vi "CommandFIFO.vi"   [LabVIEW 2018]
uses:
  <vilib>/rvi/Emulation/niFpgaGetClockAttributes.vi
  <vilib>/rvi/Emulation/niFpgaSctlEmulationGetInTimedLoop.vi
  <vilib>/rvi/Emulation/niFpgaEmulationReportErrorSimple.vi
  <vilib>/rvi/interface/RandomDataEmulation/niFpgaRandomDataHandleErrors.vi
  <vilib>/rvi/DataTransferAndStorage/Container/Common/niFpgaContainerExecOnDevCompGetState.vi
  <vilib>/rvi/Emulation/niFpgaEmulationIsFPGAContextNoSignature.vi
  <vilib>/rvi/errors/niFpgaSetErrorForExecOnDevCompSimple.vi
  <vilib>/rvi/eio/common/nirviEmuReportErrorAndStop.vi
  <vilib>/rvi/DataTransferAndStorage/Container/Common/niFpgaContainerGetUniqueNameForEmu.vi
  <vilib>/rvi/FIFO/Fifo_Resource/nirvififoEmulationSetSize.vi
  <vilib>/rvi/FIFO/Fifo_Resource/nirviFifoEmulationQueueMgr.vi
  <instcachedir>/0/nirviFifoEmulationQueueMgr_E5CAEC123FF24DC58D834DCA3CDAA9B5.lvgen/nirviFifoEmulationQueueMgr_E5CAEC123FF24DC58D834DCA3CDAA9B5_012.vi
  <vilib>/rvi/FIFO/Fifo_Resource/nirvififoEmulationDetermineInputValidOut.vi
  <vilib>/rvi/FIFO/Fifo_Resource/nirvififoEmulationCreateLock.vi
  <vilib>/rvi/Emulation/niFpgaProcessEmulError.vi
  <vilib>/rvi/FIFO/Fifo_Resource/nirvififoEmulationObtainLock.vi
  <vilib>/rvi/FIFO/Fifo_Resource/nirvififoEmulationReleaseLock.vi
  <vilib>/rvi/occurrence/nirviWaitOnOccurrenceBase.vi
  <vilib>/rvi/errors/nirviReportUnexpectedCaseInternalError.vi
  <vilib>/rvi/errors/nirviReportUnexpectedCaseInternalError (U32).vi
  <vilib>/Utility/error.llb/Clear Errors.vi
  <vilib>/rvi/Memory/Memory_Emulation/niFpgaMemoryEmulationCacheClearOnFirstRun.vi
  <vilib>/rvi/Memory/Memory_Emulation/nirvimemoryEmulationManagerCache_MakeExclusive.vi
  <vilib>/rvi/Memory/Memory_Emulation/niFpgaMemoryEmulationValidateCache.vi
  <vilib>/rvi/Memory/Memory_Emulation/nirvimemoryEmulationManagerCache_InsertValue.vi
  <vilib>/rvi/Memory/Memory_Emulation/nirvimemoryEmulationManagerCache_ReleaseExclusive.vi
  <vilib>/rvi/Memory/Memory_Emulation/nirvimemoryEmulationManagerCache_GetValue.vi
  <vilib>/rvi/Memory/Memory_Emulation/nirvimemoryEmulationManagerCache_SetValue.vi
  <instcachedir>/0/nirviFifoEmulationQueueMgr_E5CAEC123FF24DC58D834DCA3CDAA9B5.lvgen/nirviFifoEmulationQueueMgr_E5CAEC123FF24DC58D834DCA3CDAA9B5_017.vi
  <vilib>/rvi/Emulation/niFpgaCriticalErrorInLSC.vi
  <vilib>/rvi/DataTransferAndStorage/Container/XNode/niFpgaContainer.xnode
  <vilib>/rvi/interface/RandomDataEmulation/nirviRandomDataFpgaReadWriteTemplate.vi
  <vilib>/rvi/FIFO/Fifo_Resource/niFpgaFifoEmulationRefIn.vi
  <vilib>/rvi/DataTransferAndStorage/Register/Emulation/niFpgaRegisterEmulation.vi
  <vilib>/rvi/FIFO/Fifo_Resource/nirvififoEmulationWrite.vi
types:
  T1 = typedef "Addresses.ctl" = enum8{"NA", "Accelerometers", "Timestamp", "ChasisTemperature"}
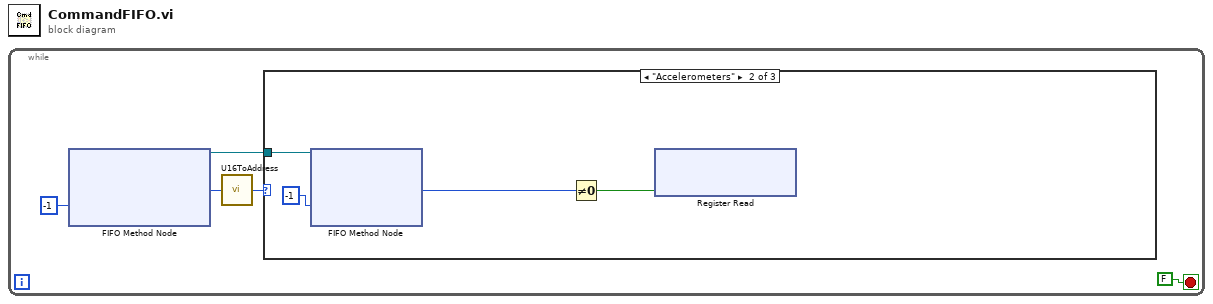
[diagram p0: block diagram]
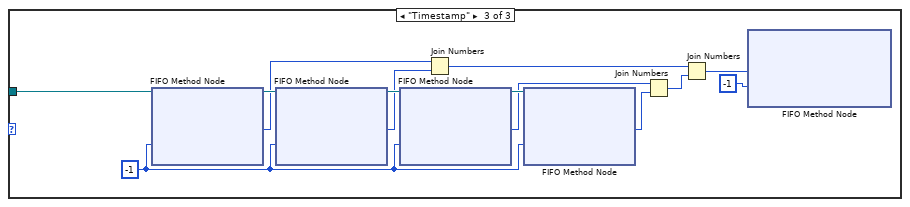
[diagram p3: hidden frame]
diagram:
  n1 = while {
    stop <- FALSE stop-if-true
    n2 = xnode ("FIFO Method Node")("Timeout"=-1) -> ("Element"=w3:u16, "FIFO Out"=w1:refnum<k21>)  [unwired: 1 in, 1 out]
    n3 = call "U16ToAddress.vi"("Input"=w3) -> ("Addresses"=w2:T1)
    n4 = case shown="\"Accelerometers\"" w2 {
      tunnel: w1 -> [_ w9 w19]
      frame "NA", Default {
      }
      frame "Accelerometers" {
        n5 = xnode ("FIFO Method Node")("Timeout"=-1, "FIFO In"=w9) -> ("Element"=w7:u16)  [unwired: 2 out]
        n6 = Not Equal To 0?(x=w7) -> (x != 0?=w6:bool)
        n7 = xnode "Register Read"("Data"=w6) -> ()  [unwired: 1 in, 1 out]
      }
      frame "Timestamp" {
        w18 = -1 ("Timeout")
        n8 = xnode ("FIFO Method Node")("Timeout"=w18, "FIFO In"=w19) -> ("Element"=w16:u16, "FIFO Out"=w22:refnum<k21>)  [unwired: 1 out]
        n9 = xnode ("FIFO Method Node")("Timeout"=w18, "FIFO In"=w22) -> ("Element"=w15:u16, "FIFO Out"=w21:refnum<k21>)  [unwired: 1 out]
        n10 = xnode ("FIFO Method Node")("Timeout"=w18, "FIFO In"=w21) -> ("Element"=w14:u16, "FIFO Out"=w20:refnum<k21>)  [unwired: 1 out]
        n11 = Join Numbers(hi=w16, lo=w15) -> ((hi.lo)=w12:u32)
        n12 = xnode ("FIFO Method Node")("Timeout"=w18, "FIFO In"=w20) -> ("Element"=w13:u16)  [unwired: 2 out]
        n13 = Join Numbers(hi=w14, lo=w13) -> ((hi.lo)=w11:u32)
        n14 = Join Numbers(hi=w12, lo=w11) -> ((hi.lo)=w10:u64)
        n15 = xnode ("FIFO Method Node")("Element"=w10, "Timeout"=-1) -> ()  [unwired: 1 in, 2 out]
      }
    }
  }
